vi "xy data storing.vi"(1 "X-ArrayStorage Input":dbl[][](array[numeric])=array1025x10[10250 elements] format="%.2f", 3 "Y-ArrayStorage Input":dbl[][](array[numeric])=array1025x10[10250 elements] format="%.2f", 4 "Pinning Input":bool[](array[boolean])=[FALSE, FALSE, FALSE, FALSE, FALSE, FALSE, FALSE, FALSE, FALSE, FALSE], 5 "File Info Storage Input":T1[](array[typedef]) {"CCD Parameters"."dt or s" format="%#.6f"; "CCD Parameters"."Repetition" min=1; "CCD Parameters"."Offset" format="%#.2f"; "CCD Parameters"."Exposure Time (s)" min=0.02 max=6000.0 format="%#.2f"; "Center nm" format="%.2f"; "Temperature (K)" format="%.2f"; "Field (T)" format="%.2f"}, 6 "xData Input":dbl[][](array[numeric])=array1025x10[10250 elements] format="%.2f", 7 "StoreInto":u16(ring) items=["Store Into", "Previous", "older", "Ref#1", "Ref#2", "Ref#3", "Ref#4", "Ref#5", "Ref#6", "Ref#7"], 10 "yData Input":dbl[][](array[numeric])=array1025x10[10250 elements] format="%.2f", 12 "File Info Input":T1[](array[typedef]) {"CCD Parameters"."dt or s" format="%#.6f"; "CCD Parameters"."Repetition" min=1; "CCD Parameters"."Offset" format="%#.2f"; "CCD Parameters"."Exposure Time (s)" min=0.02 max=6000.0 format="%#.2f"; "Center nm" format="%.2f"; "Temperature (K)" format="%.2f"; "Field (T)" format="%.2f"}) -> (9 "File Info Mixed Output":T1[](array[typedef]) {"CCD Parameters"."dt or s" format="%#.6f"; "CCD Parameters"."Repetition" min=1; "CCD Parameters"."Offset" format="%#.2f"; "CCD Parameters"."Exposure Time (s)" min=0.02 max=6000.0 format="%#.2f"; "Center nm" format="%.2f"; "Temperature (K)" format="%.2f"; "Field (T)" format="%.2f"}, 11 "xMixed Array":dbl[][](array[numeric]) format="%.2f", 13 "yMixed Array":dbl[][](array[numeric]) format="%.2f", 14 "X-ArrayStorage Output":dbl[][](array[numeric]) format="%.2f", 15 "Y-ArrayStorage Output":dbl[][](array[numeric]) format="%.2f", 16 "Pinning Output":bool[](array[boolean]), 17 "File Info Storage Output":T1[](array[typedef]) {"CCD Parameters"."dt or s" format="%#.6f"; "CCD Parameters"."Repetition" min=1; "CCD Parameters"."Offset" format="%#.2f"; "CCD Parameters"."Exposure Time (s)" min=0.02 max=6000.0 format="%#.2f"; "Center nm" format="%.2f"; "Temperature (K)" format="%.2f"; "Field (T)" format="%.2f"}, 18 "StoreInto Reset":i8)   [LabVIEW 2024]
doc: "The Array storage dimensions are 1024 x 10.\n\nIf StoreInto > 0, set the current xData & yData into the StorageRegister, which is the column where \"Pinning Input\" is true;\nAlso call xy data filter to mix the xyData with the StorageRegister"
uses:
  Globals and TypeDefs/Type Definitions.llb/FileInfoParameter.ctt
  Globals and TypeDefs/Type Definitions.llb/Wavelength Unit.ctt
  Globals and TypeDefs/Type Definitions.llb/McPherson Grating Density.ctl
  Globals and TypeDefs/Type Definitions.llb/CCDParameter.ctt
  Globals and TypeDefs/Type Definitions.llb/OperationMode.ctt
  Globals and TypeDefs/Type Definitions.llb/ListOfDetectors.ctt
panel:
  in  "Case Constant\n(See Context Help)":bool
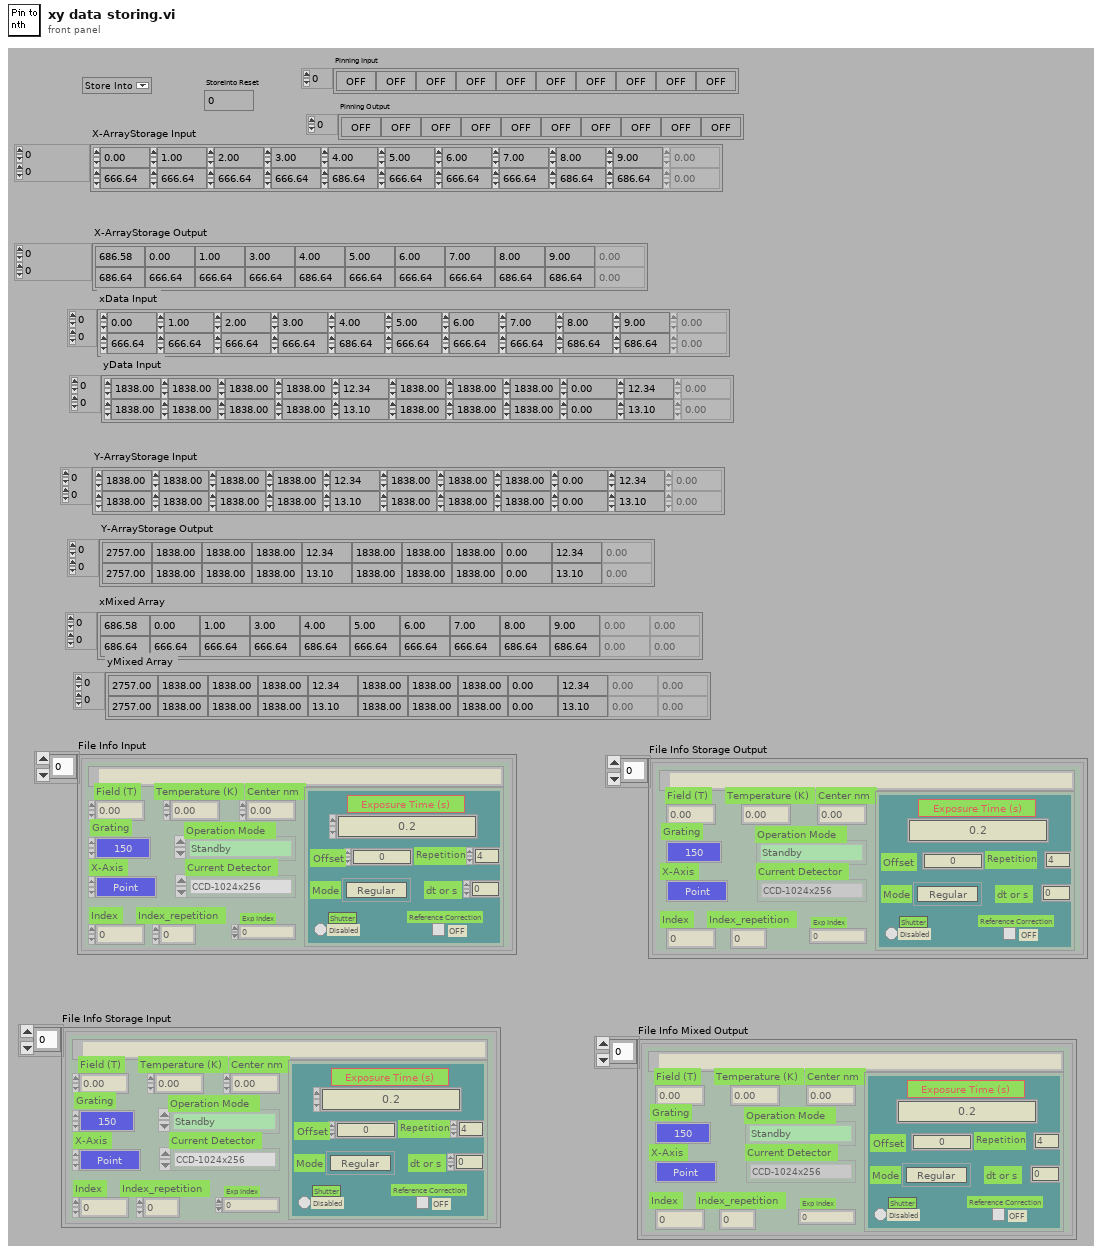
[diagram p1: front panel]
types:
  T1 = typedef "FileInfoParameter.ctt" = cluster{"FilePath":path, "Field (T)":dbl, "Temperature (K)":dbl, "X-Axis":T2, "Center nm":dbl, "Current Grating Density":T3, "CCD Parameters":T4, "Operation Mode":T5, "Exp Index":u32, "Index_repetition":u16, "Index":u16, "Current Detector":T6}
  T2 = typedef "Wavelength Unit.ctt" = enum8{"Point", "nm", "eV", "meV", "cm_1"}
  T3 = typedef "McPherson Grating Density.ctl" = enum8{"150", "300", "600", "1200", "1800"}
  T4 = typedef "CCDParameter.ctt" = cluster{"Exposure Time (s)":dbl, "Offset":dbl, "BkgrdCrct":bool, "Shutter":bool, "Mode":enum8{"Regular", "OverExp Cor", "SpikeRemove", "ForCalibration"}, "Repetition":u16, "dt or s":dbl}
  T5 = typedef "OperationMode.ctt" = enum16{"Standby", "CCD Single Shot", "CCD Sequence Shots", "CCD Custom Shots", "CCD Reference Shot", "Step Scanning ", "Time Scanning", "NML Data Acquisition"}
  T6 = typedef "ListOfDetectors.ctt" = enum8{"CCD-1024x256", "InGaAs PDA-1024x1", "CCD-1340x400", "Ge Single Channel", "Si Single Channel", "PMT Single Channel"}
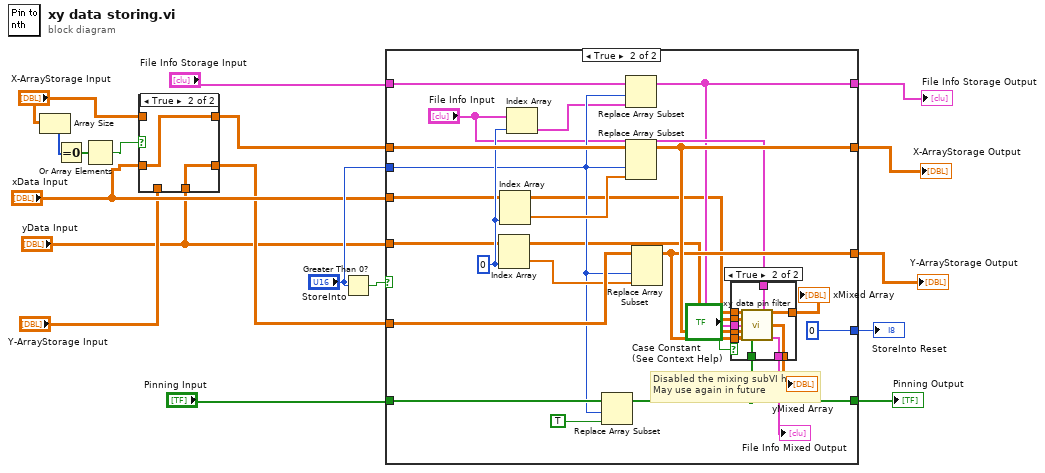
[diagram p0: block diagram]
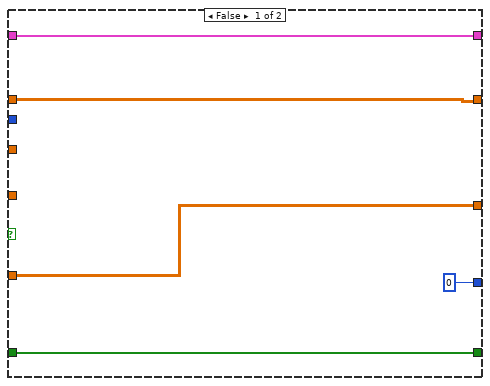
[diagram p3: hidden frame]
diagram:
  n1 = Array Size(array="X-ArrayStorage Input") -> (size(s)=w9:i32[])
  n2 = Equal To 0?(x=w9) -> (x = 0?=w8:bool[])
  n3 = Or Array Elements(Boolean array=w8) -> (logical OR=w7:bool)
  n4 = case shown="True" w7 {
    tunnel: "X-ArrayStorage Input" -> [w20 _]
    tunnel: [w20 w22] -> w5
    tunnel: "xData Input" -> [_ w22]
    tunnel: [w19 w21] -> w3
    tunnel: "Y-ArrayStorage Input" -> [w19 _]
    tunnel: "yData Input" -> [_ w21]
    frame False {
    }
    frame True {
    }
  }
  n5 = Greater Than 0?(x="StoreInto") -> (x > 0?=w18:bool)
  n6 = case shown="True" w18 {
    tunnel: w5 -> [w27 w49]
    tunnel: "StoreInto" -> [_ w35]
    tunnel: w3 -> [w25 w47]
    tunnel: [w27 w42] -> w16
    tunnel: [w25 w41] -> w15
    tunnel: [0 ("disabled index (col)") 0 ("disabled index (col)")] -> w14
    tunnel: "Pinning Input" -> [w24 w44]
    tunnel: [w24 w40] -> w12
    tunnel: "File Info Storage Input" -> [w23 w36]
    tunnel: [w23 w32] -> w10
    tunnel: "xData Input" -> [_ w29]
    tunnel: "yData Input" -> [_ w28]
    frame False {
    }
    frame True {
      w37 = 0 ("disabled index (col)")
      # "Disabled the mixing subVI here.\nMay use again in future"
      n7 = Index Array(array=w28, index (col)=w37) -> (element=w46:dbl[])  [unwired: 1 in]
      n8 = Index Array(array=w29, index (col)=w37) -> (element=w48:dbl[])  [unwired: 1 in]
      n9 = Index Array(array="File Info Input", index=w37) -> (element=w34:T1)
      n10 = Replace Array Subset(array=w44, new element=TRUE, index=w35) -> (w40:bool[])
      n11 = Replace Array Subset(array=w36, new element=w34, index=w35) -> (w32:T1[])
      n12 = Replace Array Subset(array=w49, new element=w48, index (col)=w35) -> (w42:dbl[][])  [unwired: 1 in]
      n13 = Replace Array Subset(array=w47, new element=w46, index (col)=w35) -> (w41:dbl[][])  [unwired: 1 in]
      n14 = case shown="True" "Case Constant\n(See Context Help)" {
        tunnel: w29 -> [w51 w62]
        tunnel: w28 -> [_ w61]
        tunnel: w42 -> [_ w60]
        tunnel: w41 -> [w50 w59]
        tunnel: w40 -> [_ w58]
        tunnel: [w51 w57] -> w39
        tunnel: [w50 w56] -> w38
        tunnel: "File Info Input" -> [w52 w55]
        tunnel: w32 -> [_ w54]
        tunnel: [w52 w53] -> w31
        frame False {
        }
        frame True {
          n15 = call "xy data pin filter.vi"("X-Axis Array Input"=w62, "Fixed items"=w58, "File Info Input"=w55, "Data Array Input"=w61, "File Info Old"=w54, "X-Axis Array Old"=w60, "Data Array Old"=w59) -> ("X-Axis Array output"=w57:dbl[][], "Data Array output"=w56:dbl[][], "File Info Output"=w53:T1[])  [unwired: 6 in]
        }
      }
      "xMixed Array" <- w39
      "yMixed Array" <- w38
      "File Info Mixed Output" <- w31
    }
  }
  "Y-ArrayStorage Output" <- w15
  "X-ArrayStorage Output" <- w16
  "StoreInto Reset" <- w14
  "Pinning Output" <- w12
  "File Info Storage Output" <- w10
